vi "DIAdem Enqueue Query Request.vi"(8 "error in (no error)":errorcluster, 10 "Wait for Completion?":bool=TRUE, 11 "Query Request":T2={"UserName"="", "Search Parameters"=[], "eSearch Type"=enum."eSearchFile", "Query Name (vbs)"="Spartan_Query.VBS", "Response queue name"="", "Logic String"=""}) -> (0 "error out":errorcluster, 2 "timed out?":bool, 3 "Query Data":T1)   [LabVIEW 2011]
uses:
  DataFinder/eSearch Types.ctl
  DataFinder/DataFinder Comparisons.ctl
  DataFinder/Datafinder Query.ctl
  Query Queue.ctl
  Query Result.ctl
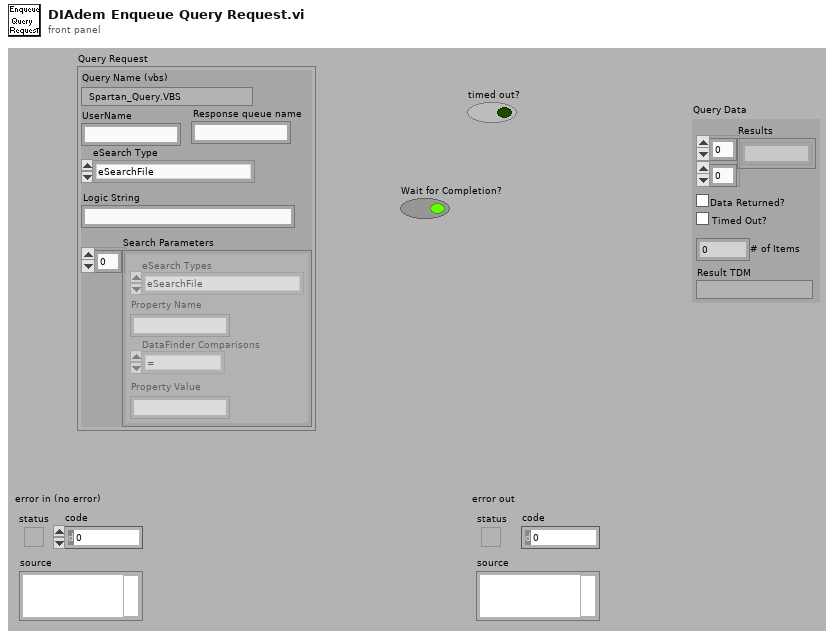
[diagram p1: front panel]
types:
  T1 = typedef "Query Result.ctl" = cluster{"Results":string[][], "# of Items":i32, "Data Returned?":bool, "Result TDM":path, "Timed Out?":bool}
  T2 = typedef "Query Queue.ctl" = cluster{"UserName":string, "Search Parameters":T3[], "eSearch Type":T4, "Query Name (vbs)":string, "Response queue name":string, "Logic String":string}
  T3 = typedef "Datafinder Query.ctl" = cluster{"eSearch Types":T4, "Property Name":string, "DataFinder Comparisons":T5, "Property Value":string}
  T4 = typedef "eSearch Types.ctl" = enum16{"eSearchFile", "eSearchChannelGroup", "eSearchChannel"}
  T5 = typedef "DataFinder Comparisons.ctl" = enum16{"=", "<>", "<", "<=", ">", ">="}
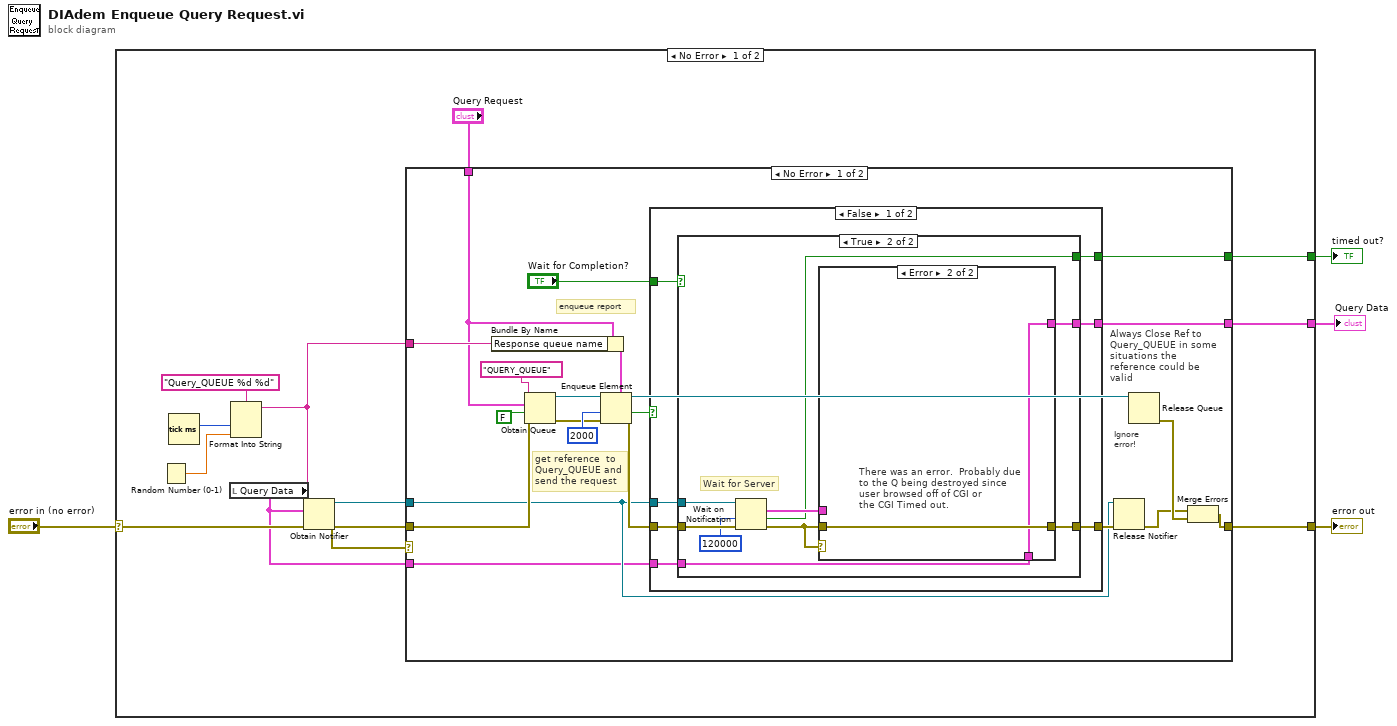
[diagram p0: block diagram]
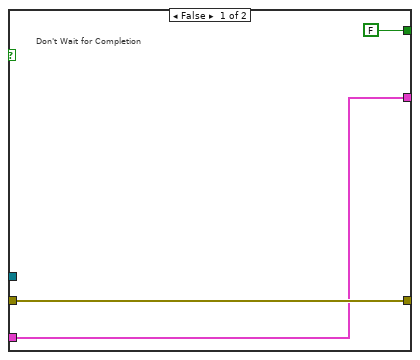
[diagram p2: hidden frame]
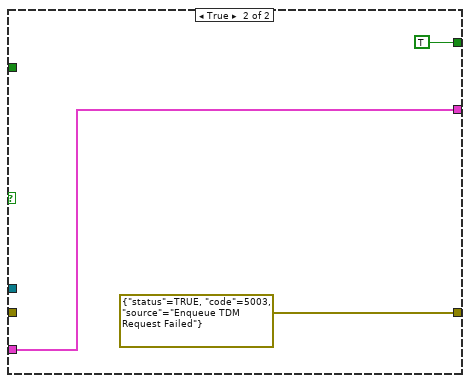
[diagram p4: hidden frame]
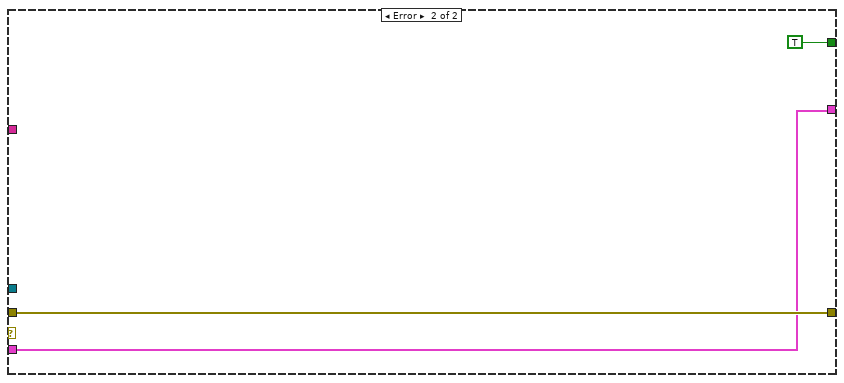
[diagram p5: hidden frame]
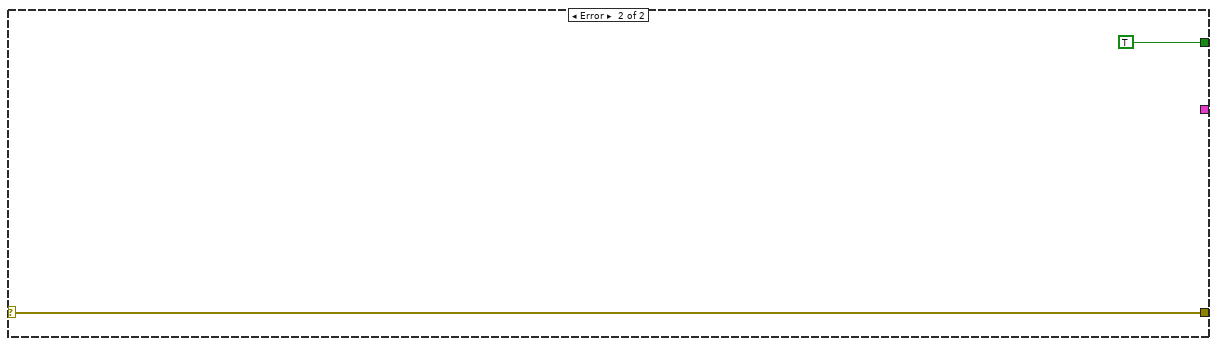
[diagram p6: hidden frame]
diagram:
  n1 = case shown="No Error" "error in (no error)" {
    selector: "error in (no error)" -> [w13 w67]
    tunnel: [w16 _] -> w1
    tunnel: [w15 w67] -> w4
    tunnel: [w14 TRUE ("timed out?")] -> w3
    frame No Error {
      n2 = Random Number (0-1)() -> (number: 0 to 1=w9:dbl)
      n3 = Tick Count (ms)() -> (millisecond timer value=w10:u32)
      n4 = local read "Query Data"() -> (w5:T1)
      n5 = Format Into String(format string="Query_QUEUE %d %d" ("name (unnamed)"), w10, w9) -> (resulting string=w7:string)  [unwired: 2 in, 1 out]
      n6 = Obtain Notifier(name (unnamed)=w7, notification data type=w5, error in (no error)=w13) -> (notifier out=w6:refnum<notifier>, error out=w8:errorcluster)  [unwired: 1 in, 1 out]
      n7 = case shown="No Error" w8 {
        tunnel: [w37 w64] -> w16
        tunnel: [w23 w66] -> w15
        tunnel: [w26 TRUE ("timed out?")] -> w14
        tunnel: w6 -> [w19 _]
        tunnel: w8 -> [w25 w66]
        tunnel: w7 -> [w22 _]
        tunnel: "Query Request" -> [w21 _]
        tunnel: w5 -> [w17 w64]
        frame No Error {
          # "Ignore\nerror!"
          # "Always Close Ref to Query_QUEUE in some situations the reference could be valid"
          # "enqueue report"
          # "get reference  to \nQuery_QUEUE and\nsend the request"
          n8 = Bundle By Name(cluster=w21, "Response queue name"=w22) -> (w36:T2)
          n9 = Obtain Queue(name (unnamed)="QUERY_QUEUE", element data type=w21, create if not found? (T)=FALSE, error in (no error)=w25) -> (queue out=w29:refnum<queue>, error out=w30:errorcluster)  [unwired: 1 in, 1 out]
          n10 = Enqueue Element(queue=w29, element=w36, timeout in ms (-1)=2000, error in (no error)=w30) -> (queue out=w33:refnum<queue>, timed out?=w31:bool, error out=w32:errorcluster)
          n11 = case shown="False" w31 {
            tunnel: w32 -> [w43 _]
            tunnel: w19 -> [w44 _]
            tunnel: [w42 errorcluster {"status"=TRUE, "code"=5003, "source"="Enqueue TDM Request Failed"} ("error out")] -> w20
            tunnel: "Wait for Completion?" -> [w41 _]
            tunnel: [w40 w61] -> w37
            tunnel: [w39 TRUE ("timed out?")] -> w26
            tunnel: w17 -> [w38 w61]
            frame False {
              n12 = case shown="True" w41 {
                tunnel: w44 -> [_ w51]
                tunnel: w43 -> [w47 w50]
                tunnel: [w47 w56] -> w42
                tunnel: [w45 w55] -> w40
                tunnel: [FALSE ("timed out?") w53] -> w39
                tunnel: w38 -> [w45 w48]
                frame False {
                  # "Don't Wait for Completion"
                }
                frame True {
                  # "Wait for Server"
                  n13 = Wait on Notification(notifier=w51, timeout in ms (-1)=120000, error in (no error)=w50) -> (notification=w54:T1, timed out?=w53:bool, error out=w52:errorcluster)  [unwired: 2 out]
                  n14 = case shown="Error" w52 {
                    tunnel: [w58 w60] -> w56
                    tunnel: [w57 w59] -> w55
                    tunnel: w54 -> [w57 _]
                    tunnel: w52 -> [w58 w60]
                    tunnel: w48 -> [_ w59]
                    frame No Error {
                    }
                    frame Error {
                      # "There was an error.  Probably due\nto the Q being destroyed since\nuser browsed off of CGI or\nthe CGI Timed out."
                    }
                  }
                }
              }
            }
            frame True {
            }
          }
          n15 = Release Notifier(notifier=w19, error in (no error)=w20) -> (error out=w18:errorcluster)  [unwired: 3 out]
          n16 = Release Queue(queue=w33) -> (error out=w24:errorcluster)  [unwired: 1 in, 3 out]
          n17 = Merge Errors(w18, w24) -> (w23:errorcluster)
        }
        frame Error {
        }
      }
    }
    frame Error {
    }
  }
  "timed out?" <- w3
  "error out" <- w4
  "Query Data" <- w1
